vi "SMU2450Init.vi"(6 "Keithley Config":T1={"Source Compliance (A)"=0.1, "Min Voltage (V)"=0.0, "Max Voltage (V)"=5.0, "Source Mode"=0, "Number of Points"=50} {"Number of Points" min=2 step=1; "Source Mode" items=["Voltage", "Current"]; "Min Voltage (V)" min=0.1}, 8 "error in (no error)":errorcluster, 11 "Keithley 2400 Name":refnum<visa-resource-name>) -> (0 "error out":errorcluster, 3 "VISA resource name out":refnum<visa-resource-name>)   [LabVIEW 2019, in "SMU.lvclass"]
uses:
  SMU.lvclass
  typeDefs/keithleySettings.ctl
panel:
  out "concatenated string":string
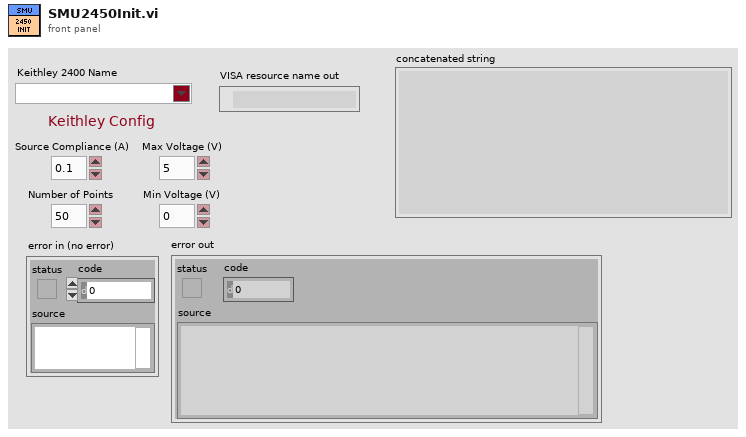
[diagram p1: front panel]
types:
  T1 = typedef "keithleySettings.ctl" = cluster{"Source Compliance (A)":dbl, "Min Voltage (V)":dbl, "Max Voltage (V)":dbl, "Source Mode":u16, "Number of Points":u32}
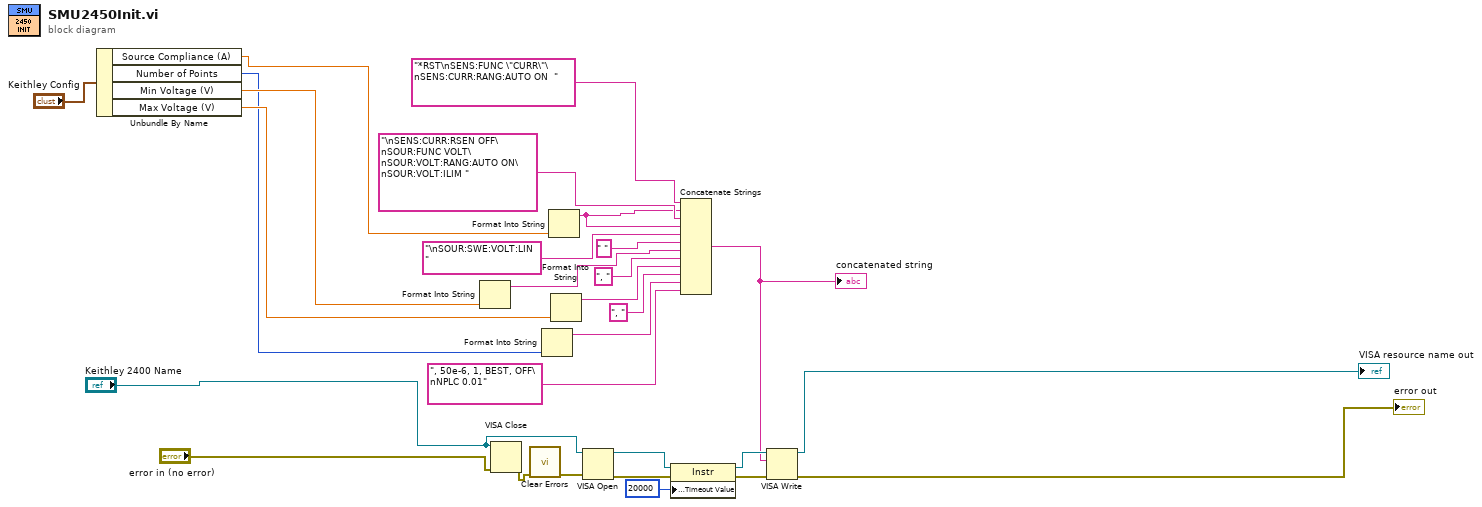
[diagram p0: block diagram]
diagram:
  n1 = Unbundle By Name("Keithley Config") -> ("Source Compliance (A)"=w23:dbl, "Number of Points"=w20:u32, "Min Voltage (V)"=w22:dbl, "Max Voltage (V)"=w21:dbl)
  n2 = Format Into String(w22) -> (resulting string=w16:string)  [unwired: 3 in, 1 out]
  n3 = VISA Close(VISA resource name="Keithley 2400 Name", error in (no error)="error in (no error)") -> (error out=w6:errorcluster)
  n4 = call <vilib>:"Clear Errors.vi"("error in (no error)"=w6) -> ("error out"=w1:errorcluster)  [unwired: 5 in, 1 out]
  n5 = Format Into String(w20) -> (resulting string=w14:string)  [unwired: 3 in, 1 out]
  n6 = Format Into String(w23) -> (resulting string=w3:string)  [unwired: 3 in, 1 out]
  n7 = Format Into String(w21) -> (resulting string=w5:string)  [unwired: 3 in, 1 out]
  n8 = VISA Open(error in (no error)=w1, VISA resource name="Keithley 2400 Name") -> (VISA resource name=w9:refnum<visa-resource-name>, error out=w11:errorcluster)  [unwired: 3 in]
  n9 = property class="Instr"(reference=w9, error in=w11, "General Settings:Timeout Value"=u32 20000) -> (reference out=w8:refnum<visa-resource-name>, error out=w10:errorcluster)
  n10 = Concatenate Strings("*RST\nSENS:FUNC \"CURR\"\nSENS:CURR:RANG:AUTO ON  " ("write buffer"), w3, "\nSENS:CURR:RSEN OFF\nSOUR:FUNC VOLT\nSOUR:VOLT:RANG:AUTO ON\nSOUR:VOLT:ILIM ", w3, "\nSOUR:SWE:VOLT:LIN ", " " ("string"), w16, ", " ("string"), w5, ", " ("string"), w14, ", 50e-6, 1, BEST, OFF\nNPLC 0.01") -> (w7:string)
  "concatenated string" <- w7
  n11 = VISA Write(VISA resource name=w8, write buffer=w7, error in (no error)=w10) -> (VISA resource name out=→"VISA resource name out":refnum<visa-resource-name>, error out=→"error out":errorcluster)  [unwired: 1 out]
